vi "Graph - XY-03788.vi"() -> ()   [LabVIEW 2014]
doc: "Sample numeric display item."
uses:
  <vilib>/NI Veristand/Display Template Support/Display Template Support.llb/cluster_Screen Item Settings.ctl
  <vilib>/NI Veristand/Display Template Support/Display Template Support.llb/cluster_Graph Scale Settings.ctl
  <vilib>/NI Veristand/Display Template Support/Display Template Support.llb/cluster_Graph Plot Settings.ctl
  <vilib>/NI Veristand/Display Template Support/Display Template Support.llb/cluster_Graph Handler Message.ctl
  <vilib>/NI Veristand/Display Template Support/Display Template Support.llb/enum_Graph Handler Message.ctl
  <vilib>/NI Veristand/Display Template Support/Display Template Support.llb/sub_Display Template Data Handler Graph.vi
  <vilib>/NI Veristand/Display Template Support/Display Template Support.llb/sub_Display Template Handler Graph.vi
panel:
  out "XY Graph":cluster{dbl[], dbl[]}(graph)
  out "Graph":waveform(dbl)[](graph)
  out "Label":string="Numeric"
  out "Y.Autoscale":bool
  in  "Y.Scale.Auto":bool
  out "X.Autoscale":bool
  in  "X.Scale.Auto":bool
  in  "Legend":bool
  in  "Setup":bool
  in  "Hold":bool
  in  "Item.Data":T1
  # "Autoscale X"
  # "Autoscale Y"
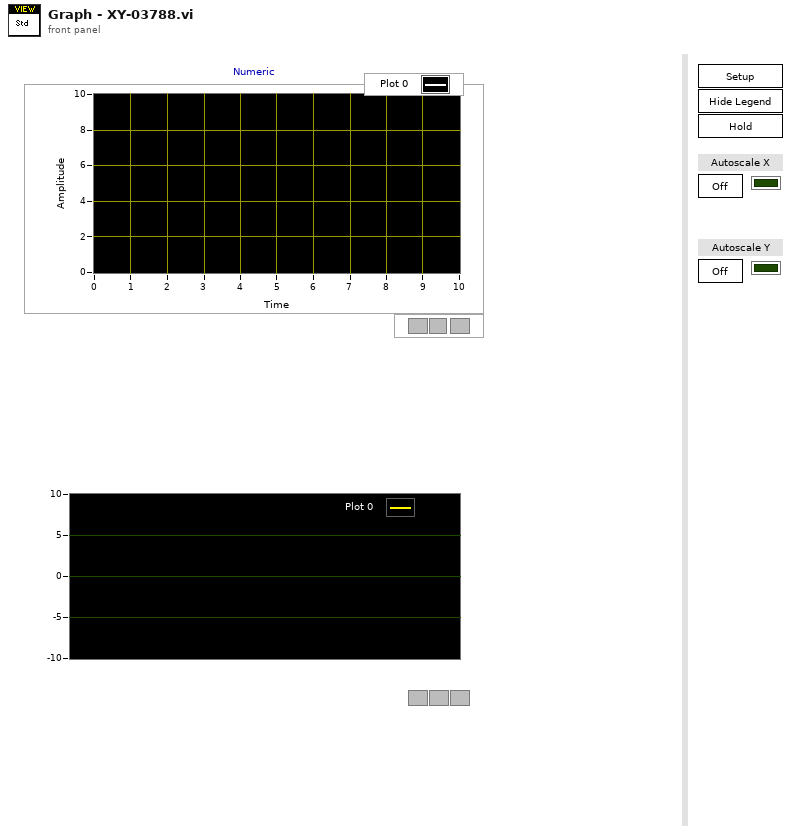
[diagram p1: front panel]
types:
  T1 = typedef "cluster_Screen Item Settings.ctl" = cluster{"Template VI":string, "Position X":i32, "Position Y":i32, "Custom":string, "Show Title Bar":bool, "ID":i32, "Always On Top":bool, "Allow Resize":bool, "Allow Minimize":bool, "Allow Close":bool, "Size to Screen":bool, "Screen.ID":i32, "State":enum16{"Normal", "New"}, "Title":string, "Window Bounds":cluster{"[0]":i16, "[1]":i16, "[2]":i16, "[3]":i16}, "Channel Ref":u64, "Unit":string, "Default Units?":bool, "Flash Limit?":bool, "Color 1":u32, "Color 2":u32, "Color 3":u32, "Color 4":u32, "Bck Color":u32, "Fore Color":u32, "Limit 1":dbl, "Limit 2":dbl, "Limit 3":dbl, "Limit 4":dbl, "Limit Mode 1":i32, "Limit Mode 2":i32, "Limit Mode 3":i32, "Limit Mode 4":i32, "Scale Precision":i32, "Scale Min":dbl, "Scale Max":dbl, "Format":i32, "Precision":i32, "Background Type":i32, "IDs":i32[], "Units":string[], "Labels":string[], "Scale Factor":dbl, "Scale Offset":dbl, "YScale Index":u32[], "XScale":T2, "YScales":T2[], "Plots":T3[], "Update Period":dbl, "History Length":dbl, "My.Ref":refnum<vi>, "Is Control?":bool, "Channel Paths":string[], "Custom Data":variant}
  T2 = typedef "cluster_Graph Scale Settings.ctl" = cluster{"Format":u8, "Precision":u8, "Fit":u8, "Label":string, "Use Default Label":bool, "Label Visible":bool, "Min":dbl, "Max":dbl}
  T3 = typedef "cluster_Graph Plot Settings.ctl" = cluster{"Bar Style":u8, "Fill To":i16, "Fill/PtColor":u32, "Line Style":u8, "Line Width":u8, "Color":u32, "Interp":u8, "Point Style":u8}
  T4 = typedef "cluster_Graph Handler Message.ctl" = cluster{"Message":T5, "Data":variant}
  T5 = typedef "enum_Graph Handler Message.ctl" = enum16{"None", "Stop", "Hold", "Update Channels", "New Settings", "Control Value", "Edit Value"}
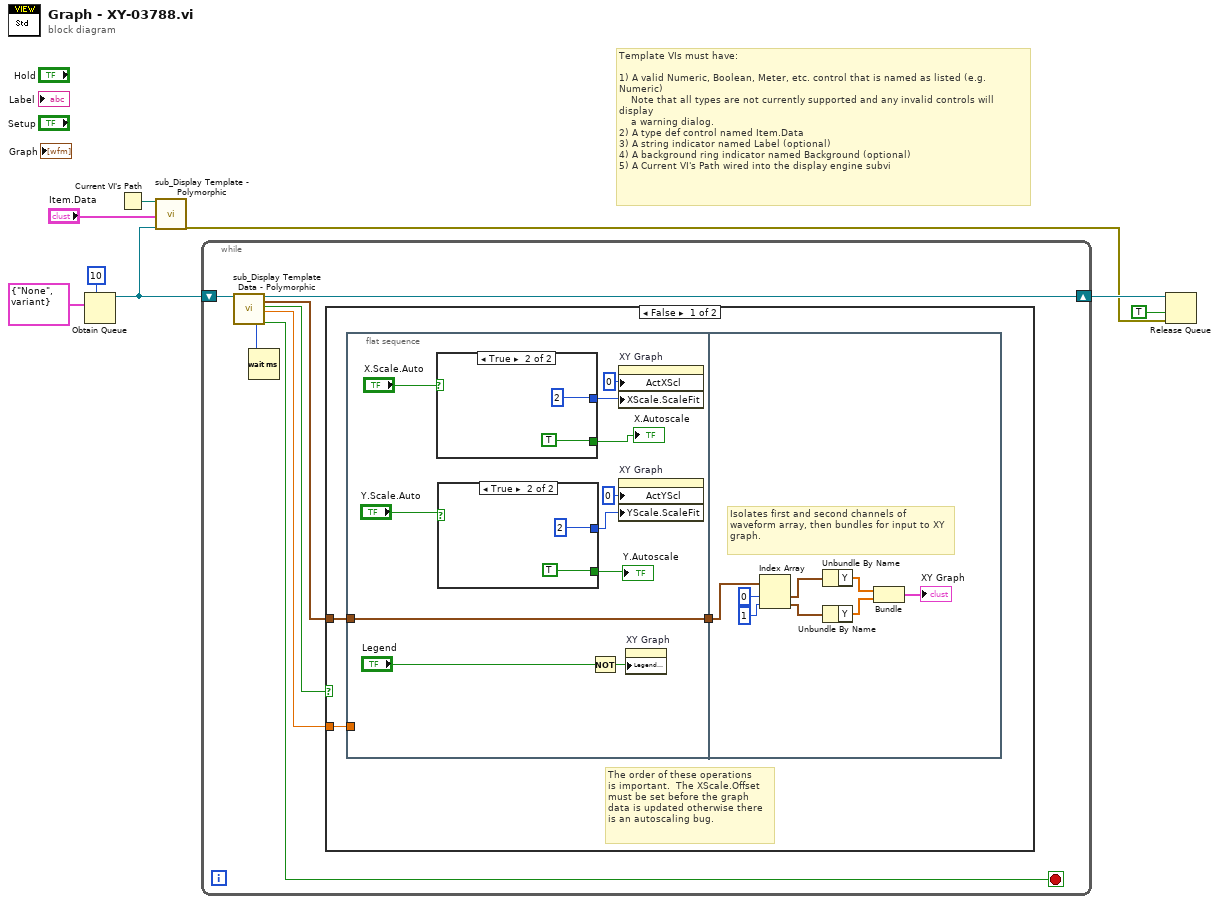
[diagram p0: block diagram]
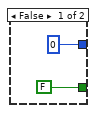
[diagram p2: hidden frame]
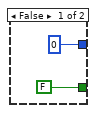
[diagram p3: hidden frame]
diagram:
  # "Template VIs must have:\n\n1) A valid Numeric, Boolean, Meter, etc. control that is named as listed (e.g. Numeric)\n    Note that all types are not currently supported and any invalid controls will display\n    a warning dialog.\n2) A type def control named Item.Data\n3) A string indicator named Label (optional)\n4) A background ring indicator named Background (optional)\n5) A Current VI's Path wired into the display engine subvi"
  n1 = Obtain Queue(max queue size (-1, unlimited)=10, element data type=T4 {"Message"=enum."None", "Data"=variant} ("Message")) -> (queue out=w2:refnum<queue>)  [unwired: 2 in, 3 out]
  n2 = Current VI's Path() -> (path=w8:path)
  n3 = call-poly <vilib>:"sub_Display Template - Polymorphic.vi"("Parent.Path"=w8, "Item.Data"="Item.Data", "queue"=w2) -> ("error out"=w1:errorcluster)  [unwired: 16 out]
  n4 = while {
    shift-right: [w15] -> w6
    shift-left: w2 -> [w14]
    stop <- w9 stop-if-true
    n5 = call-poly <vilib>:"sub_Display Template Data - Polymorphic.vi"("queue"=w14) -> ("Wait.Time"=w12:u32, "queue out"=w15:refnum<queue>, "Graph.Data"=w13:waveform(dbl)[], "Hold"=w10:bool, "XScale.Offset"=w11:dbl, "Stop"=w9:bool)  [unwired: 13 out]
    n6 = Wait (ms)(milliseconds to wait=w12) -> ()  [unwired: 1 out]
    n7 = case shown="False" w10 {
      tunnel: w11 -> [w18 _]
      tunnel: w13 -> [w17 _]
      frame False {
        # "The order of these operations\nis important.  The XScale.Offset\nmust be set before the graph\ndata is updated otherwise there\nis an autoscaling bug."
        n8 = flat-sequence {
          tunnel: w18 -> [_]
          tunnel: w17 -> [w29]
          tunnel: [w29] -> w16
          tunnel: w16 -> [w43]
          frame #0 {
            n9 = case shown="True" "X.Scale.Auto" {
              tunnel: [FALSE TRUE] -> w24
              tunnel: [u8 0 ("X Scale.Scale Fit") u8 2 ("X Scale.Scale Fit")] -> w23
              frame False {
              }
              frame True {
              }
            }
            "X.Autoscale" <- w24
            n10 = case shown="True" "Y.Scale.Auto" {
              tunnel: [FALSE TRUE] -> w19
              tunnel: [u8 0 ("X Scale.Scale Fit") u8 2 ("X Scale.Scale Fit")] -> w21
              frame False {
              }
              frame True {
              }
            }
            "Y.Autoscale" <- w19
            n11 = Not(x="Legend") -> (.not. x?=w28:bool)
            n12 = property on="XY Graph" class="XYGraph (strict)"("ActXScl"=0 ("Active X Scale"), "XScale.ScaleFit"=w23) -> ()  [unwired: 2 in, 2 out]
            n13 = property on="XY Graph" class="XYGraph (strict)"("ActYScl"=0 ("Active X Scale"), "YScale.ScaleFit"=w21) -> ()  [unwired: 2 in, 2 out]
            n14 = property on="XY Graph" class="XYGraph (strict)"("Legend Visible"=w28) -> ()  [unwired: 2 in, 2 out]
          }
          frame #1 {
            # "Isolates first and second channels of waveform array, then bundles for input to XY graph."
            n15 = Index Array(array=w43, index #1=0 ("index"), index #2=1 ("index")) -> (element #1=w42:waveform(dbl), element #2=w41:waveform(dbl))
            n16 = Unbundle By Name(w42) -> ("Y"=w40:dbl[])
            n17 = Unbundle By Name(w41) -> ("Y"=w39:dbl[])
            n18 = Bundle("Y"=w40, "Y"=w39) -> (→"XY Graph":cluster{"Y":dbl[], "Y":dbl[]})  [unwired: 1 in]
          }
        }
      }
      frame True {
      }
    }
  }
  n19 = Release Queue(queue=w6, force destroy? (F)=TRUE, error in (no error)=w1) -> ()  [unwired: 3 out]
